vi "initialiseFields.vi"(8 "error in (no error)":errorcluster, 11 "ScanCreator in":refnum<class "ScanCreator.lvclass">) -> (0 "error out":errorcluster, 3 "ScanCreator out":refnum<class "ScanCreator.lvclass">)   [LabVIEW 2009, in "Views.lvlib" / "ScriptEditor.lvlib" / "ScanCreator.lvclass"]
uses:
  ScanCreator.lvclass
  ScanCreator.lvclass/ScanCreator.ctl
  Tools/Scripting/ScriptingEvent/ScriptEvent.lvclass
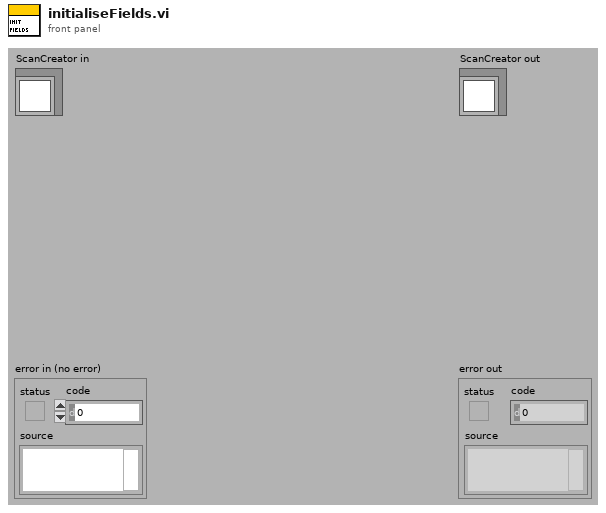
[diagram p1: front panel]
types:
  T1 = enum16{"changeValue", "pulse", "clock", "rampUp", "rampDown", "singleTone", "singleToneRamp", "playFile", "rf", "rfRamp"}
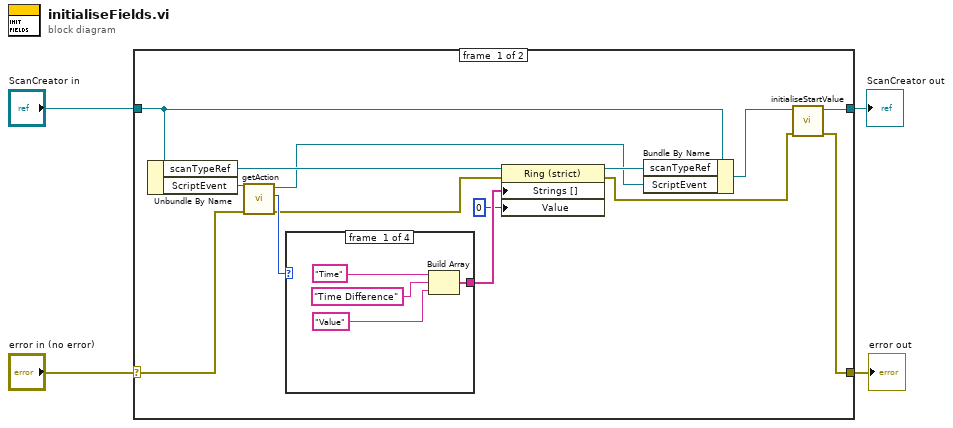
[diagram p0: block diagram]
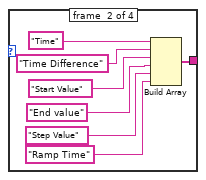
[diagram p2: hidden frame]
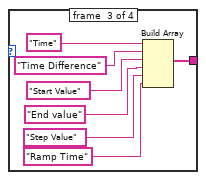
[diagram p3: hidden frame]
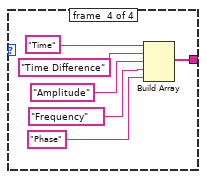
[diagram p4: hidden frame]
diagram:
  n1 = case shown="No Error" "error in (no error)" {
    selector: "error in (no error)" -> [w17 w44]
    tunnel: [w11 w44] -> w3
    tunnel: [w12 w43] -> w1
    tunnel: "ScanCreator in" -> [w10 w43]
    frame #0 {
      n2 = Unbundle By Name(w10) -> ("scanTypeRef"=w15:refnum<vi>, "ScriptEvent"=w18:refnum<class "ScriptEvent.lvclass">)
      n3 = call "getAction.vi"("error in (no error)"=w17, "ScriptEvent.lvclass in"=w18) -> ("error out"=w13:errorcluster, "action"=w16:T1, "ScriptEvent.lvclass out"=w8:refnum<class "ScriptEvent.lvclass">)  [unwired: 7 in]
      n4 = case shown="\"changeValue\", Default" w16 {
        tunnel: [w19 w28 w31 w37] -> w14
        frame #0 {
          n5 = Build Array("Time", "Time Difference", "Value") -> (w19:string[])
        }
        frame #1 {
          n6 = Build Array("Time", "Time Difference", "Start Value", "End value", "Step Value", "Ramp Time") -> (w28:string[])
        }
        frame #2 {
          n7 = Build Array("Time", "Time Difference", "Start Value", "End value", "Step Value", "Ramp Time") -> (w31:string[])
        }
        frame #3 {
          n8 = Build Array("Time", "Time Difference", "Amplitude", "Frequency", "Phase") -> (w37:string[])
        }
      }
      n9 = property class="Ring (strict)"(reference=w15, error in=w13, "Strings []"=w14, "Value"=0) -> (reference out=w9:refnum<vi>, error out=w7:errorcluster)
      n10 = Bundle By Name(cluster=w10, "scanTypeRef"=w9, "ScriptEvent"=w8) -> (w6:refnum<class "ScanCreator.lvclass">)
      n11 = call "initialiseStartValue.vi"("error in (no error)"=w7, "ScanCreator in"=w6) -> ("error out"=w11:errorcluster, "ScanCreator out"=w12:refnum<class "ScanCreator.lvclass">)  [unwired: 8 in]
    }
    frame #1 {
    }
  }
  "error out" <- w3
  "ScanCreator out" <- w1
